vi "7.99.1-Blinky Light Lookup Table Values.vi"() -> (0 "Init Data Out":u8[](array[numeric]))   [LabVIEW 2010]
doc: "This VI runs on the Dev Computer, and it generates a lookup table for the Blinky Light PWM."
panel:
  in  "Full period Magnitude":i16=100
  in  "First Harmonic Magnitude":i16=40
  in  "Second Harmonic Magnitude":i16=70
  out "Waveform Graph":u8[](graph)
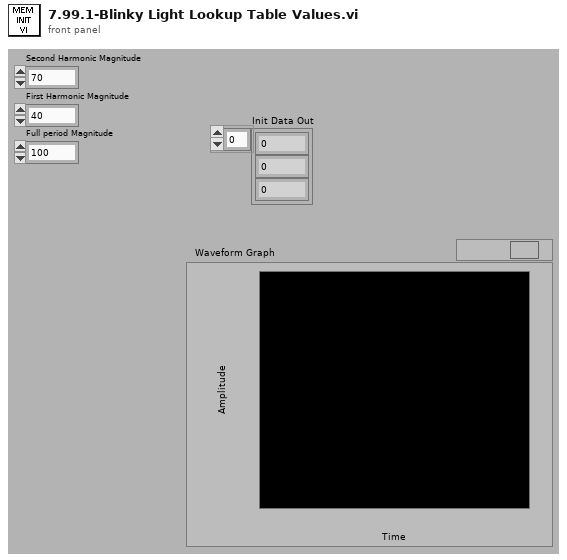
[diagram p1: front panel]
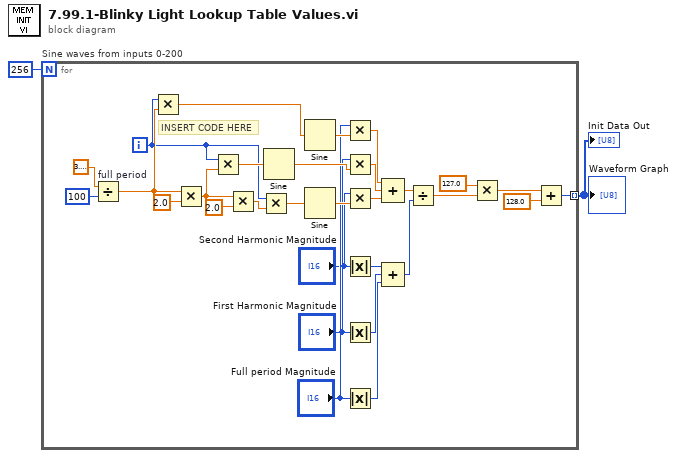
[diagram p0: block diagram]
diagram:
  n1 = for "Sine waves from inputs 0-200" {
    N: u32 256 -> [_]
    tunnel: [w10] -> w1 mode=indexing
    i -> [w6]
    # "INSERT CODE HERE"
    n2 = Divide "full period"(x=3.141592653589793, y=100) -> (x/y=w28:dbl)
    n3 = Multiply(x=w6, y=w28) -> (x*y=w9:dbl)
    n4 = Multiply(x=w28, y=2.0) -> (x*y=w27:dbl)
    n5 = Multiply(x=w6, y=w27) -> (x*y=w8:dbl)
    n6 = Multiply(x=w27, y=2.0) -> (x*y=w26:dbl)
    n7 = Multiply(x=w6, y=w26) -> (x*y=w7:dbl)
    n8 = Sine(x=w8) -> (sin(x)=w21:dbl)
    n9 = Sine(x=w9) -> (sin(x)=w22:dbl)
    n10 = Sine(x=w7) -> (sin(x)=w20:dbl)
    n11 = Multiply(x="Full period Magnitude", y=w22) -> (x*y=w23:dbl)
    n12 = Multiply(x="First Harmonic Magnitude", y=w21) -> (x*y=w24:dbl)
    n13 = Multiply(x="Second Harmonic Magnitude", y=w20) -> (x*y=w25:dbl)
    n14 = Absolute Value(x="Second Harmonic Magnitude") -> (abs(x)=w5:i16)
    n15 = Absolute Value(x="First Harmonic Magnitude") -> (abs(x)=w3:i16)
    n16 = Absolute Value(x="Full period Magnitude") -> (abs(x)=w4:i16)
    n17 = Compound Arithmetic op=ADD(w23, w24, w25) -> (w16:dbl)
    n18 = Compound Arithmetic op=ADD(w5, w3, w4) -> (w15:i16)
    n19 = Divide(x=w16, y=w15) -> (x/y=w14:dbl)
    n20 = Multiply(x=127.0, y=w14) -> (x*y=w12:dbl)
    n21 = Add(x=w12, y=128.0) -> (x+y=w10:u8)
  }
  "Init Data Out" <- w1
  "Waveform Graph" <- w1
